vi "Get Files By Extension.vi"(8 "Error In":errorcluster, 10 "Extention":string, 11 "Directory":path) -> (0 "Error Out":errorcluster, 3 "Files With Extension":path[](array[path]))   [LabVIEW 2014, in "LMH-Toolbox.lvlib"]
doc: "This VI returns all of the files within the specicied directory that have the specified file extension."
uses:
  <vilib>/MakerHub/Toolbox/LMH-Toolbox.lvlib
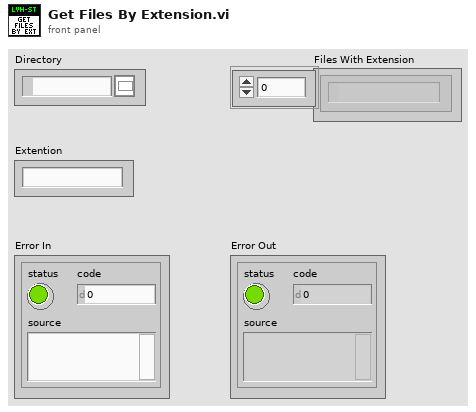
[diagram p1: front panel]
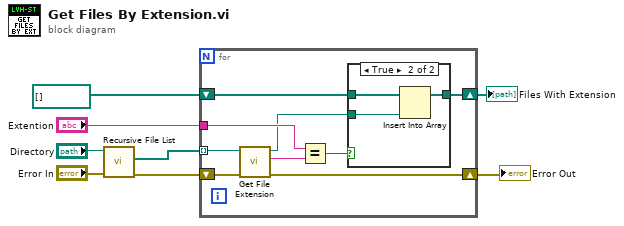
[diagram p0: block diagram]
diagram:
  n1 = call <vilib>:"Recursive File List.vi"("error in (no error)"="Error In", "Folder Path"="Directory") -> ("error out"=w4:errorcluster, "All Files in Dir"=w6:path[])  [unwired: 5 in, 3 out]
  n2 = for {
    tunnel: w6 -> [w17] mode=indexing
    tunnel: "Extention" -> [w14]
    shift-right: [w13] -> w3
    shift-left: w4 -> [w16]
    shift-right: [w9] -> w1
    shift-left: path[] [] -> [w12]
    n3 = call <vilib>:"Get File Extension.vi"("Error In"=w16, "File Path Control"=w17) -> ("Error Out"=w13:errorcluster, "Extension"=w15:string, "Duplicate Path"=w11:path)  [unwired: 7 in]
    n4 = Equal?(x=w14, y=w15) -> (x = y?=w10:bool)
    n5 = case shown="True" w10 {
      tunnel: w12 -> [w18 w21]
      tunnel: w11 -> [_ w20]
      tunnel: [w18 w19] -> w9
      frame False {
      }
      frame True {
        n6 = Insert Into Array(array=w21, new element=w20) -> (w19:path[])  [unwired: 1 in]
      }
    }
  }
  "Error Out" <- w3
  "Files With Extension" <- w1
